vi "TouchScreen.vi"() -> ()   [LabVIEW 2018]
uses:
  <vilib>/Platform/TimedLoop/XDataNode/timing_clust.ctl
  <vilib>/Platform/TimedLoop/XDataNode/nitl_modes.ctl
  <vilib>/Platform/TimedLoop/XDataNode/wakeup.ctl
  <vilib>/rvi/Emulation/niFpgaSctlEmulationGetInTimedLoop.vi
  <vilib>/rvi/Emulation/niFpgaEmulationReportErrorSimple.vi
  <vilib>/rvi/Emulation/niFpgaGetClockAttributes.vi
  <vilib>/rvi/Emulation/niFpgaCriticalErrorInLSC.vi
  <vilib>/rvi/eio/common/nirviEmuTemplateMethod_errors.vi
  <vilib>/Platform/TimedLoop/XDataNode/XDataNode.xnode
  <vilib>/eio/EIONode/EIONode.xnode
  <vilib>/Platform/TimedLoop/XDataNode/XDNodeRunTimeDep.lvlib
  Downloads/LabVIEW DSDB Examples/LabVIEW DSDB Examples/Shared Library/I2C/I2C FPGA.lvlib
panel:
  in  "TFT_DIM":u16=5
  in  "I2C.DataOut":u8
  in  "I2C.GO":bool
  in  "I2C.Control":u8
  in  "I2C.Address":u8
  in  "I2C.Counter":u16=187
  out "I2C.DataIn":u8
  out "I2C.Status":u8
  in  "I2C.Configuration":u8
  in  "radius":fxp<+,8,8>
  in  "TFT_Reset":bool=TRUE
  in  "TFT_Display":bool=TRUE
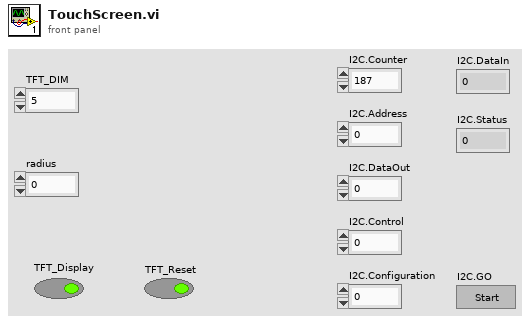
[diagram p1: front panel]
types:
  T1 = typedef "XDNodeRunTimeDep.lvlib/timing_clust.ctl" = cluster{"Expected End [f-1]":u64, "Actual End [f-1]":u64, "Finished Late? [f-1]":bool, "Expected End [i-1]":u64, "Actual End [i-1]":u64, "Finished Late? [i-1]":bool, "Expected Start [i]":u64, "Actual Start [i]":u64, "Expected Start [f]":u64, "Actual Start [f]":u64, "Source Name":string, "Structure Name":string, "Period":i64, "Deadline":i64, "Offset":i64, "Start":i64, "Priority":i32, "Timeout":i32, "Mode":T2, "Wakeup Reason":T3, "Error":errorcluster, "Source Type":string, "Secondary Source Type":string, "Global End Time":u64, "Global Start Time":u64, "Frame Duration":u64, "Iteration Duration":u64, "Assigned CPU":i32, "I/O Scan Engine Mode":u32}
  T2 = typedef "XDNodeRunTimeDep.lvlib/nitl_modes.ctl" = enum32{"No Change", "Process missed periods, maintain original phase", "Discard missed periods, maintain original phase", "Process missed periods, ignore original phase", "Discard missed periods, ignore original phase"}
  T3 = typedef "XDNodeRunTimeDep.lvlib/wakeup.ctl" = enum32{"Normal", "Aborted", "Asynchronous wakeup", "Timing source error", "Timed loop error", "Timeout"}
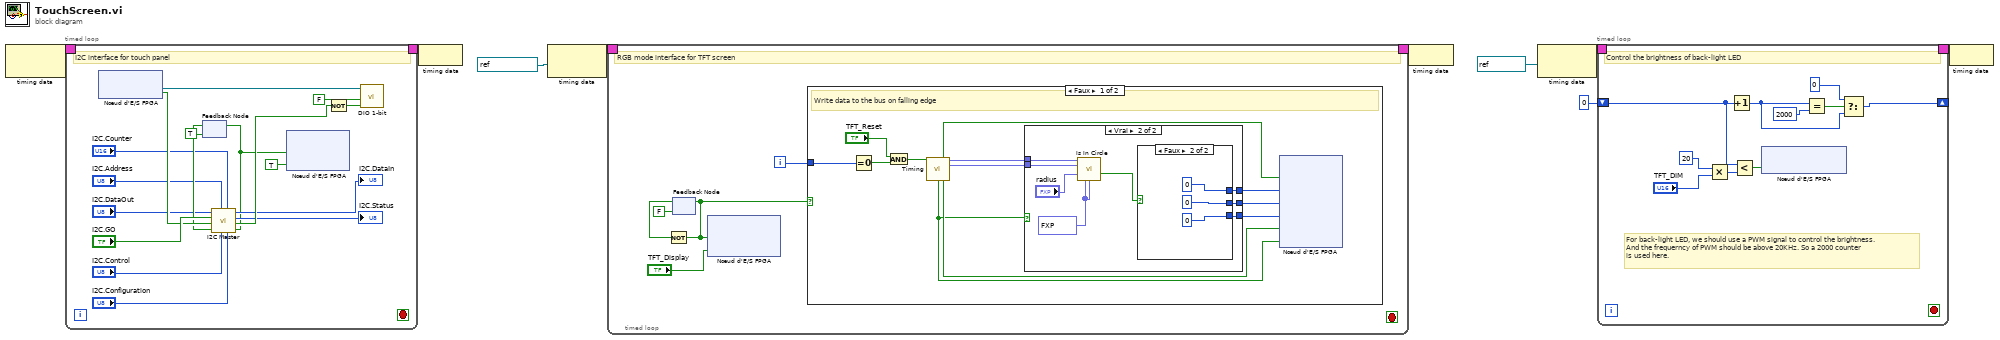
[diagram p0: block diagram]
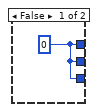
[diagram p2: hidden frame]
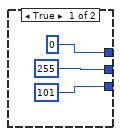
[diagram p3: hidden frame]
diagram:
  n1 = node-c288() -> (w7:T1)  [unwired: 1 in]
  n2 = timed-loop {
    timing: w7 -> [_]
    timing-out: [_] -> w6
    stop <- _ stop-if-true
    # "I2C interface for touch panel"
    n3 = xnode "Nœud d'E/S FPGA"() -> ("TP_SDA"=w21:bool, "E/S FPGA en sortie"=w12:refnum<k21>)  [unwired: 1 in]
    n4 = feedback #1(TRUE ("SCL_OUT")) -> (w20:bool)
    n5 = call "I2C Master.vi"("Configuration"="I2C.Configuration", "Counter"="I2C.Counter", "Control"="I2C.Control", "Address In"="I2C.Address", "SCL_IN"=w20, "SDA_IN"=w21, "Execute?"="I2C.GO", "Data Out"="I2C.DataOut") -> ("SCL_OUT"=w11:bool, "SDA_OUT"=w23:bool, "Status"=→"I2C.Status":u8, "Data In"=→"I2C.DataIn":u8)
    n6 = feedback-in #1(w11) -> ()
    n7 = xnode "Nœud d'E/S FPGA"("TP_SCK"=w11, "TP_RES"=TRUE) -> ()  [unwired: 2 in, 2 out]
    n8 = Not(x=w23) -> (.not. x?=w24:bool)
    n9 = call "DIO 1-bit.vi"("DIR"=w24, "OUT"=FALSE, "DIO Refnum"=w12) -> ()  [unwired: 8 in, 1 out]
  }
  n10 = node-c288(w6) -> ()
  n11 = node-c288(refnum<k21> "71,68MHz" ("Source Name")) -> (w9:T1)
  n12 = timed-loop {
    timing: w9 -> [_]
    timing-out: [_] -> w8
    i -> [w31]
    stop <- _ stop-if-true
    # "RGB mode interface for TFT screen"
    n13 = feedback #2(FALSE) -> (w32:bool)
    n14 = Not(x=w32) -> (.not. x?=w30:bool)
    n15 = feedback-in #2(w30) -> ()
    n16 = xnode "Nœud d'E/S FPGA"("TFT_DCLK"=w30, "TFT_DISP"="TFT_Display") -> ()  [unwired: 2 in, 2 out]
    n17 = case shown="Faux" w30 {
      tunnel: w31 -> [w45 _]
      frame False {
        # "Write data to the bus on falling edge"
        n18 = Equal To 0?(x=w45) -> (x = 0?=w37:bool)
        n19 = And(x="TFT_Reset", y=w37) -> (x .and. y?=w39:bool)
        n20 = call "Timing.vi"("Reset"=w39) -> ("HSync"=w36:bool, "HPixel"=w41:fxp<+,10,10>, "VPixel"=w40:fxp<+,10,10>, "DE"=w34:bool, "VSync"=w35:bool)  [unwired: 10 in]
        n21 = case shown="Vrai" w34 {
          tunnel: w41 -> [_ w51]
          tunnel: w40 -> [_ w50]
          tunnel: [w46 w54] -> w43
          tunnel: [w46 w53] -> w44
          tunnel: [w46 w52] -> w42
          frame False {
            w46 = u8 0 ("TFT_R")
          }
          frame True {
            w47 = fxp<+,12,12>[] [0.0, 0.0, 0.0, 0.0, 0.0] ("row")
            n22 = call "Is In Circle.vi"("pixel column"=w51, "pixel row"=w50, "radius"="radius", "row"=w47, "column"=w47) -> ("In Radius?"=w48:bool)  [unwired: 10 in]
            n23 = case shown="Faux" w48 {
              tunnel: [u8 255 ("TFT_G") u8 0 ("TFT_G")] -> w54
              tunnel: [u8 101 ("TFT_B") u8 0 ("TFT_B")] -> w53
              tunnel: [u8 0 ("TFT_R") u8 0 ("TFT_R")] -> w52
              frame True {
              }
              frame False {
              }
            }
          }
        }
        n24 = xnode "Nœud d'E/S FPGA"("TFT_HS"=w36, "TFT_R"=w42, "TFT_G"=w43, "TFT_B"=w44, "TFT_VS"=w35, "TFT_DE"=w34) -> ()  [unwired: 6 in, 6 out]
      }
      frame True {
        # "Screen will read data on raising edge."
      }
    }
  }
  n25 = node-c288(w8) -> ()
  n26 = node-c288(refnum<k21> "40MHz" ("Source Name")) -> (w5:T1)
  n27 = timed-loop {
    timing: w5 -> [_]
    timing-out: [_] -> w4
    shift-right: [w64] -> _
    shift-left: u16 0 -> [w65]
    stop <- _ stop-if-true
    # "For back-light LED, we should use a PWM signal to control the brightness.\nAnd the frequerncy of PWM should be above 20KHz. So a 2000 counter\nis used here."
    # "Control the brightness of back-light LED"
    n28 = Multiply(x=u16 20, y="TFT_DIM") -> (x*y=w68:u16)
    n29 = Increment(x=w65) -> (x+1=w66:u16)
    n30 = Less?(x=w65, y=w68) -> (x < y?=w69:bool)
    n31 = xnode "Nœud d'E/S FPGA"("TFT_BCKDIM"=w69) -> ()  [unwired: 1 in, 1 out]
    n32 = Equal?(x=w66, y=u16 2000) -> (x = y?=w71:bool)
    n33 = Select(t=u16 0, s=w71, f=w66) -> (s? t:f=w64:u16)
  }
  n34 = node-c288(w4) -> ()
